vi "986x.Create.vi"(8 "error in (no error)":errorcluster, 10 "986x Support":T2, 11 "Device Item Ref in":T1 format="%.0x") -> (0 "error out":errorcluster, 3 "Device Ref out":T1 format="%.0x")   [LabVIEW 2015, in "Diagnostics Addon System Explorer.lvlib"]
uses:
  Diagnostics Addon System Explorer.lvlib
  <vilib>/NI Veristand/Custom Device API/Custom Device Item Ref.ctl
  Shared/Types/986x.ctl
  <vilib>/NI/NI VeriStand SysDef Utilities/SysDef API/SysDef.Property.Remove.vi
  <vilib>/NI/NI VeriStand SysDef Utilities/_SubVIs/SysDef.Property.Set.DependentFile.vi
  <vilib>/Utility/MD5Checksum.llb/MD5Checksum File.vi
  Shared/SubVIs/Constants.vi
  <vilib>/NI/NI VeriStand SysDef Utilities/_SubVIs/SysDef.Property.Set.U16.vi
  <vilib>/NI/NI VeriStand SysDef Utilities/_SubVIs/SysDef.Property.Set.Boolean.vi
  Shared/Diagnostics Addon Shared.lvlib
  <vilib>/NI/NI VeriStand SysDef Utilities/System Definition Utilities.lvlib
  <vilib>/NI VeriStand/Custom Device API/Custom Device API.lvlib
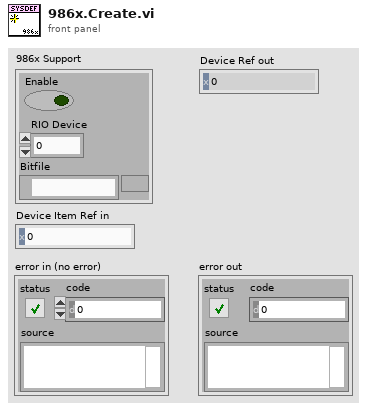
[diagram p1: front panel]
types:
  T1 = typedef "Custom Device API.lvlib/Custom Device Item Ref.ctl" = u64
  T2 = typedef "Diagnostics Addon Shared.lvlib/986x.ctl" = cluster{"Enable":bool, "RIO Device":u16, "Bitfile":path}
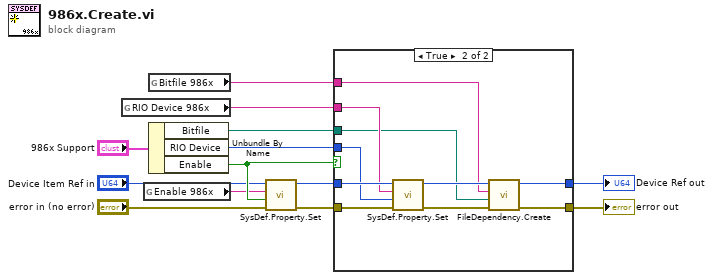
[diagram p0: block diagram]
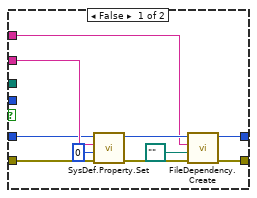
[diagram p2: hidden frame]
diagram:
  n1 = global read "Constants.vi" "RIO Device 986x"() -> (w12:string)
  n2 = global read "Constants.vi" "Enable 986x"() -> (w2:string)
  n3 = global read "Constants.vi" "Bitfile 986x"() -> (w1:string)
  n4 = Unbundle By Name("986x Support") -> ("Bitfile"=w13:path, "RIO Device"=w11:u16, "Enable"=w10:bool)
  n5 = call-poly <vilib>:"SysDef.Property.Set.vi"("error in (no error)"="error in (no error)", "Value"=w10, "Property Name"=w2, "nodeID"="Device Item Ref in") -> ("error out"=w6:errorcluster, "nodeID out"=w8:u64)  [unwired: 6 in]
  n6 = case shown="True" w10 {
    tunnel: w6 -> [w21 w33]
    tunnel: [w18 w28] -> w7
    tunnel: w8 -> [w20 w32]
    tunnel: w12 -> [w23 w30]
    tunnel: [w17 w26] -> w9
    tunnel: w11 -> [_ w31]
    tunnel: w13 -> [_ w25]
    tunnel: w1 -> [w14 w24]
    frame False {
      n7 = call-poly <vilib>:"SysDef.Property.Set.vi"("error in (no error)"=w21, "Value"=u16 0, "Property Name"=w23, "nodeID"=w20) -> ("error out"=w19:errorcluster, "nodeID out"=w16:u64)  [unwired: 6 in]
      n8 = call "FileDependency.Create.vi"("error in (no error)"=w19, "DLL Path"=path "" ("Value"), "DLL Property Name"=w14, "Item Ref in"=w16) -> ("error out"=w18:errorcluster, "Item Ref out"=w17:T1)  [unwired: 6 in]
    }
    frame True {
      n9 = call-poly <vilib>:"SysDef.Property.Set.vi"("error in (no error)"=w33, "Value"=w31, "Property Name"=w30, "nodeID"=w32) -> ("error out"=w29:errorcluster, "nodeID out"=w27:u64)  [unwired: 6 in]
      n10 = call "FileDependency.Create.vi"("error in (no error)"=w29, "DLL Path"=w25, "DLL Property Name"=w24, "Item Ref in"=w27) -> ("error out"=w28:errorcluster, "Item Ref out"=w26:T1)  [unwired: 6 in]
    }
  }
  "Device Ref out" <- w9
  "error out" <- w7
